vi "Enable UI.vi"(8 "error in (no error)":errorcluster, 11 "UI in":refnum<class "UI.lvclass">) -> (0 "error out":errorcluster, 3 "UI out":refnum<class "UI.lvclass">)   [LabVIEW 2016, in "Generic UI Actor.lvlib" / "UI.lvclass"]
uses:
  <userlib>/Common Components/User Interface/UI.lvclass
  <userlib>/Common Components/User Interface/UI.lvclass/UI.ctl
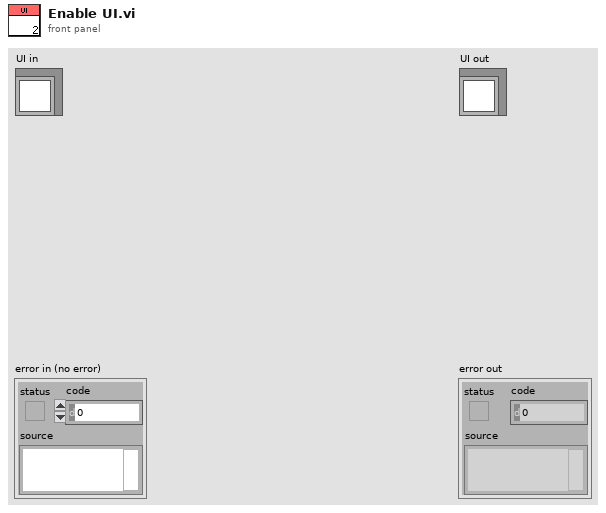
[diagram p1: front panel]
types:
  T1 = enum8{"Enabled", "Disabled", "Disabled and Grayed Out"}
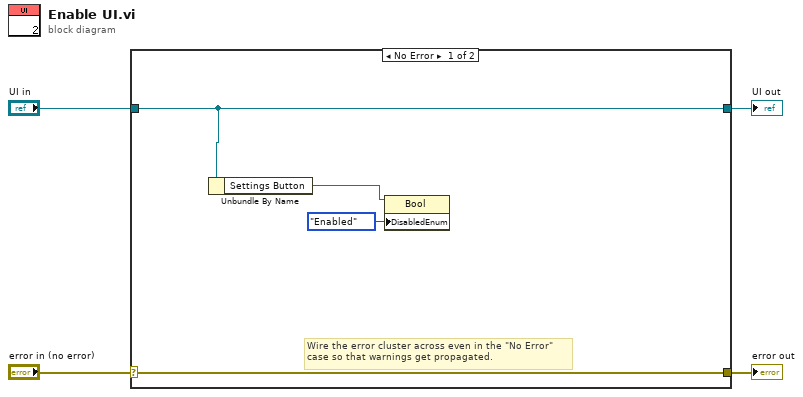
[diagram p0: block diagram]
diagram:
  n1 = case shown="No Error" "error in (no error)" {
    selector: "error in (no error)" -> [w8 w10]
    tunnel: [w8 w10] -> w3
    tunnel: [w5 w9] -> w1
    tunnel: "UI in" -> [w5 w9]
    frame No Error {
      # "Wire the error cluster across even in the \"No Error\"\ncase so that warnings get propagated."
      n2 = Unbundle By Name(w5) -> ("Settings Button"=w7:refnum<vi>)
      n3 = property class="Bool"(reference=w7, "DisabledEnum"=T1."Enabled" ("Disabled")) -> ()  [unwired: 1 in, 2 out]
    }
    frame Error {
    }
  }
  "error out" <- w3
  "UI out" <- w1
